vi "EditorInterface.vi"() -> ()   [LabVIEW 2025]
uses:
  2025RobotCode/2025ReefBot/NewAuto/NewAutoStepTypedef.ctl
  2025RobotCode/2025ReefBot/NewAuto/NewAutoStepTypeEnum.ctl
  <vilib>/Rock Robotics/WPI/ThirdParty/JAS_Junk/TrajLib/Trajectory_Library.lvlib
panel:
  in  "Write JSON":bool
  in  "DispParmNotes":bool
  in  "write":bool
  in  "read":bool
  in  "Comment":string
  in  "Path":path
  in  "Array":T1[](array[typedef])
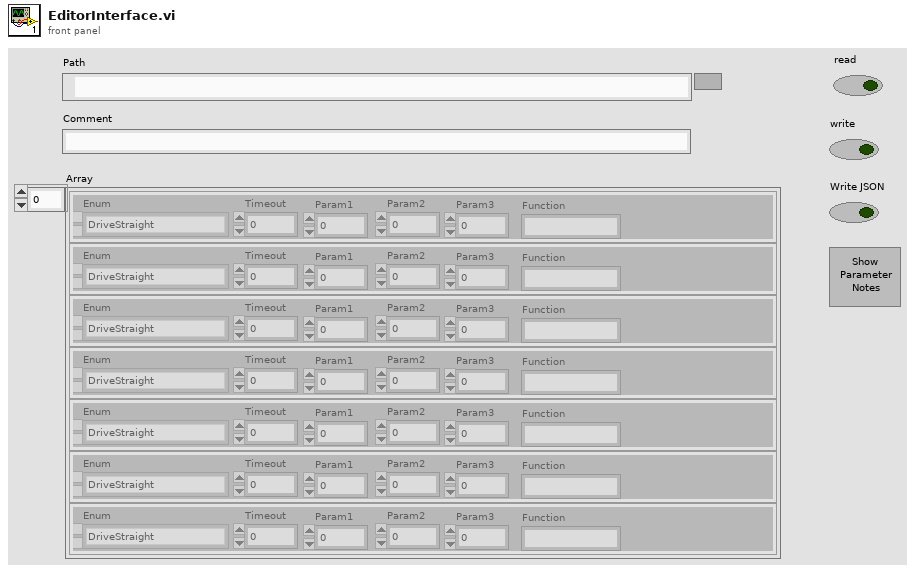
[diagram p1: front panel]
types:
  T1 = typedef "NewAutoStepTypedef.ctl" = cluster{"Enum":T2, "Timeout":dbl, "Param1":dbl, "Param2":dbl, "Param3":dbl, "Function":string}
  T2 = typedef "NewAutoStepTypeEnum.ctl" = enum16{"DriveStraight", "DriveTurn", "FollowAbsoluteTrajectory", "FollowRelativeTrajectory", "AutoWait", "FollowAbsTrajWithTimedCmd", "FollowRelTrajWithTimedComd", "Collect", "Shoot", "Stop", "BallsToAlliance", "Climb", "Descend", "Defense"}
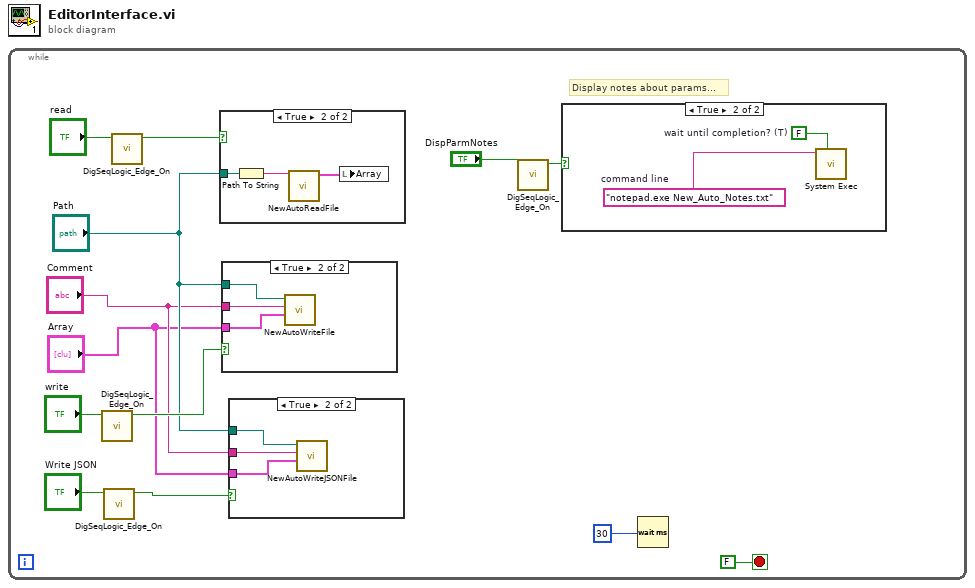
[diagram p0: block diagram]
diagram:
  n1 = while {
    stop <- FALSE stop-if-true
    # "Display notes about params..."
    n2 = call <vilib>:"DigSeqLogic_Edge_On.vi"("Input"="write") -> ("On Edge"=w11:bool)  [unwired: 10 in]
    n3 = call <vilib>:"DigSeqLogic_Edge_On.vi"("Input"="Write JSON") -> ("On Edge"=w4:bool)  [unwired: 10 in]
    n4 = call <vilib>:"DigSeqLogic_Edge_On.vi"("Input"="read") -> ("On Edge"=w12:bool)  [unwired: 10 in]
    n5 = case shown="True" w12 {
      tunnel: "Path" -> [_ w23]
      frame False {
      }
      frame True {
        n6 = Path To String(path=w23) -> (string=w22:string)
        n7 = call "NewAutoReadFile.vi"("FileName"=w22) -> ("outTRAJECTORY"=w24:T1[])  [unwired: 8 in, 2 out]
        n8 = local write "Array"(w24) -> ()
      }
    }
    n9 = case shown="True" w11 {
      tunnel: "Array" -> [_ w21]
      tunnel: "Comment" -> [_ w20]
      tunnel: "Path" -> [_ w19]
      frame False {
      }
      frame True {
        n10 = call "NewAutoWriteFile.vi"("Array"=w21, "Comment"=w20, "Trajectory File Name"=w19) -> ()  [unwired: 8 in, 1 out]
      }
    }
    n11 = case shown="True" w4 {
      tunnel: "Array" -> [_ w15]
      tunnel: "Comment" -> [_ w14]
      tunnel: "Path" -> [_ w16]
      frame False {
      }
      frame True {
        n12 = call "NewAutoWriteJSONFile.vi"("Array"=w15, "Comment"=w14, "Trajectory File Name"=w16) -> ()  [unwired: 8 in, 1 out]
      }
    }
    n13 = call <vilib>:"DigSeqLogic_Edge_On.vi"("Input"="DispParmNotes") -> ("On Edge"=w6:bool)  [unwired: 10 in]
    n14 = case shown="True" w6 {
      frame False {
      }
      frame True {
        w17 = "notepad.exe New_Auto_Notes.txt"  # command line
        w18 = FALSE  # wait until completion? (T)
        n15 = call <vilib>:"System Exec.vi"("wait until completion? (T)"=w18, "command line"=w17) -> ()  [unwired: 6 in, 4 out]
      }
    }
    n16 = Wait (ms)(milliseconds to wait=u32 30 ("millisecond timer value")) -> ()  [unwired: 1 out]
  }
